vi "Start Audio Device.vi"(8 "error in (no error)":errorcluster, 11 "Audio Device Refnum In":refnum<file>) -> (0 "error out":errorcluster, 3 "Audio Device Refnum Out":refnum<file>)   [LabVIEW 2020, in "G-Audio.lvlib"]
doc: "Start the audio device playback or capture."
uses:
  G-Audio.lvlib
  <vilib>/Utility/error.llb/Error Cluster From Error Code.vi
  lib/g_audio_x86.dll
  lib/g_audio_x64.dll
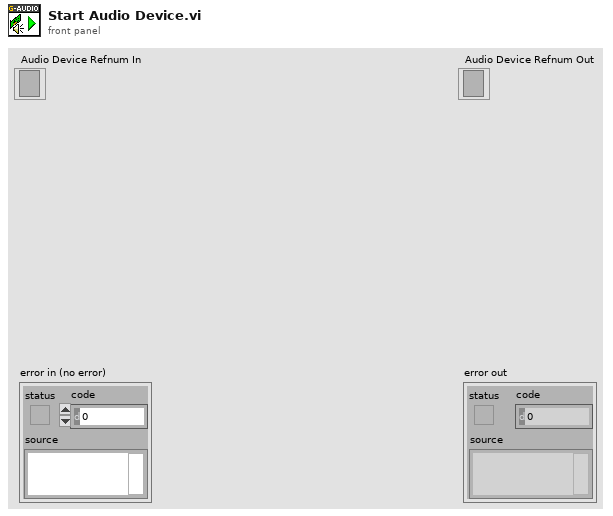
[diagram p1: front panel]
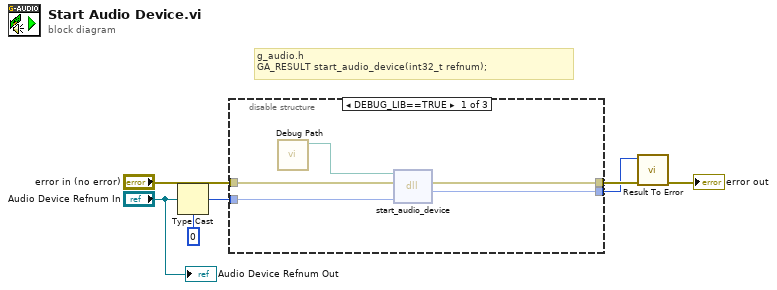
[diagram p0: block diagram]
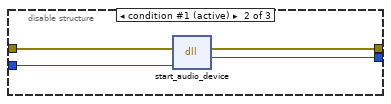
[diagram p2: hidden frame]
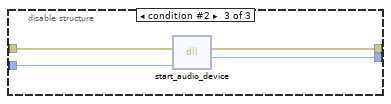
[diagram p3: hidden frame]
diagram:
  # "g_audio.h\nGA_RESULT start_audio_device(int32_t refnum);"
  n1 = Type Cast(type=0, x="Audio Device Refnum In") -> (*(type *) &x=w2:i32)
  n2 = disable-structure shown="DEBUG_LIB==TRUE" {
    disable-tunnel: "error in (no error)" -> [w9 w14 w18]
    disable-tunnel: [w11 w16 w20] -> w6
    disable-tunnel: [w10 w15 w19] -> w4
    disable-tunnel: w2 -> [w8 w13 w17]
    frame condition #0 {
      n3 = call "Debug Path.vi"() -> ("Debug Path"=w12:path)  [unwired: 11 in]
      n4 = dll-call lib="?" fn="start_audio_device"(path in=w12, error in=w9, "refnum"=w8) -> (error out=w11:errorcluster, "result"=w10:i32)  [unwired: 2 in, 1 out]
    }
    frame condition #1 (active) {
      n5 = dll-call lib="C:/github/dataflowg/g-audio/src/LabVIEW/G-Audio/lib/g_audio_x86.*" fn="start_audio_device"(error in=w14, "refnum"=w13) -> (error out=w16:errorcluster, "result"=w15:i32)  [unwired: 3 in, 1 out]
    }
    frame condition #2 {
      n6 = dll-call lib="C:/github/dataflowg/g-audio/src/LabVIEW/G-Audio/lib/g_audio_x64.*" fn="start_audio_device"(error in=w18, "refnum"=w17) -> (error out=w20:errorcluster, "result"=w19:i32)  [unwired: 3 in, 1 out]
    }
  }
  n7 = call "Result To Error.vi"("error in (no error)"=w6, "Result Code"=w4) -> ("error out"=→"error out":errorcluster)  [unwired: 9 in]
  "Audio Device Refnum Out" <- "Audio Device Refnum In"
